vi "Error Test Number Of Bits.vi"(6 "error text in":string, 8 "error in":errorcluster, 10 "number of bits":i32) -> (0 "error out":errorcluster)   [LabVIEW 2024]
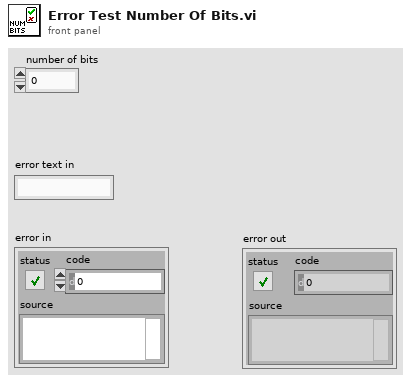
[diagram p1: front panel]
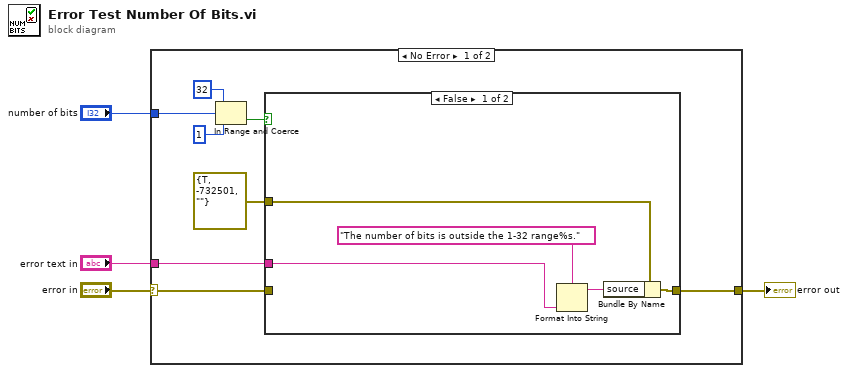
[diagram p0: block diagram]
diagram:
  n1 = case shown="No Error" "error in" {
    selector: "error in" -> [w11 w19]
    tunnel: [w10 w19] -> w3
    tunnel: "number of bits" -> [w12 _]
    tunnel: "error text in" -> [w5 _]
    frame No Error {
      n2 = In Range and Coerce(upper limit=32 ("lower limit"), x=w12, lower limit=1) -> (In Range?=w6:bool)  [unwired: 1 out]
      n3 = case shown="False" w6 {
        tunnel: w11 -> [_ w18]
        tunnel: [w16 w18] -> w10
        tunnel: errorcluster {"status"=TRUE, "code"=-732501, "source"=""} ("error constant") -> [w17 _]
        tunnel: w5 -> [w15 _]
        frame False {
          n4 = Format Into String(format string="The number of bits is outside the 1-32 range%s." ("source"), w15) -> (resulting string=w13:string)  [unwired: 2 in, 1 out]
          n5 = Bundle By Name(cluster=w17, "source"=w13) -> (w16:errorcluster)
        }
        frame True {
        }
      }
    }
    frame Error {
    }
  }
  "error out" <- w3
